vi "XYZThetaGo.vi"(8 "error in (no error)":errorcluster, 10 "XYZTheta In":dbl[](array[numeric]), 11 "Gantry In":refnum<k24>) -> (0 "error out":errorcluster, 2 "XYZTheta Out":dbl[](array[numeric]), 3 "Gantry Out":refnum<k24>)   [LabVIEW 2020, in "Motion.lvclass"]
uses:
  Motion.lvclass
  C:/Program Files (x86)/Aerotech/A3200/LabVIEW/2010/Bin/Aerotech.A3200.dll
  Program Files (x86)/Aerotech/A3200/LabVIEW/2010/Bin/Aerotech.A3200.dll
  A3200/A3200.lvclass
  Drivers/Aerotech A3200/Aerotech.lvlib
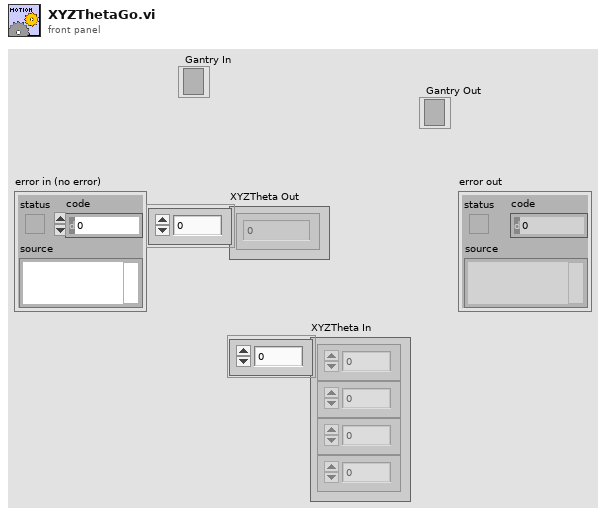
[diagram p1: front panel]
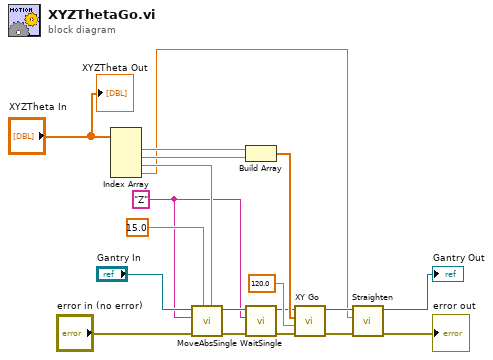
[diagram p0: block diagram]
diagram:
  w6 = "Z" ("axis name")
  n1 = Index Array(array="XYZTheta In") -> (element #1=w15:dbl, element #2=w14:dbl, element #3=w12:dbl, element #4=w1:dbl)  [unwired: 4 in]
  n2 = call "MoveAbsSingle.vi"("position"=w12, "speed"=15.0, "error in (no error)"="error in (no error)", "axis name"=w6, "controller in"="Gantry In") -> ("error out"=w4:errorcluster, "controller out"=w9:refnum<k24>)  [unwired: 5 in]
  n3 = Build Array(w15, w14) -> (w16:dbl[])
  n4 = call "WaitSingle.vi"("error in (no error)"=w4, "axis name"=w6, "controller in"=w9) -> ("error out"=w3:errorcluster, "controller out"=w8:refnum<k24>)  [unwired: 6 in, 1 out]
  n5 = call "XY Go.vi"("error in (no error)"=w3, "Speed"=120.0, "XY"=w16, "Gantry In"=w8) -> ("error out"=w13:errorcluster, "Gantry Out"=w17:refnum<k24>)  [unwired: 6 in]
  n6 = call "Straighten.vi"("error in (no error)"=w13, "Angle (rad)"=w1, "Gantry In"=w17) -> ("error out"=→"error out":errorcluster, "Gantry Out"=→"Gantry Out":refnum<k24>)  [unwired: 7 in]
  "XYZTheta Out" <- "XYZTheta In"
